vi "Particle Detection.vi"() -> ()   [LabVIEW 2014]
uses:
  <vilib>/userdefined/High Color/IMAQdx.ctl
  <vilib>/vision/driver/NI_Vision_Acquisition_Software.lvlib
  <vilib>/vision/NI_Vision_Development_Module.lvlib
panel:
  out "Before erosion":T1(plugin-control)
  out "Number of Particles after":i32
  out "After erosions":T1(plugin-control)
  in  "milliseconds to wait":u32
  out "Original":T1(plugin-control)
  in  "Number of Erosion":i32=2
  out "Number of Particles before":i32
  in  "stop":bool
  out "error out":errorcluster
  in  "error in (no error)":errorcluster
  in  "Image Name":string="webcam"
  in  "Session In":T2="cam0"
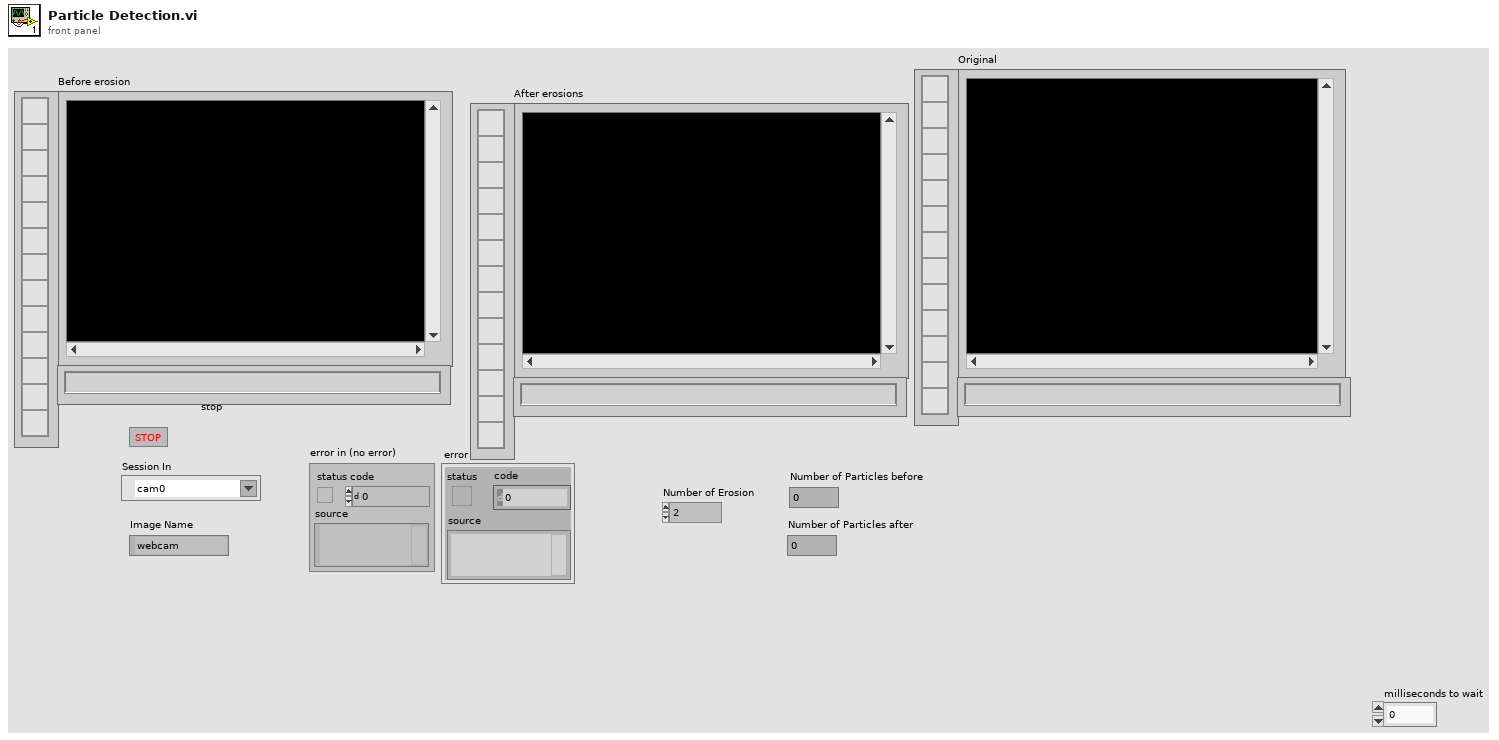
[diagram p1: front panel]
types:
  T1 = typedef "IMAQ Image.ctl" = refnum<image>
  T2 = typedef "IMAQdx.ctl" = refnum<k21>
  T3 = typedef "Image Type" = u32
  T4 = typedef "Particle Parameters" = i32
  T5 = cluster{"Numeric":dbl, "Numeric":dbl, "Numeric":dbl, "Numeric":dbl}
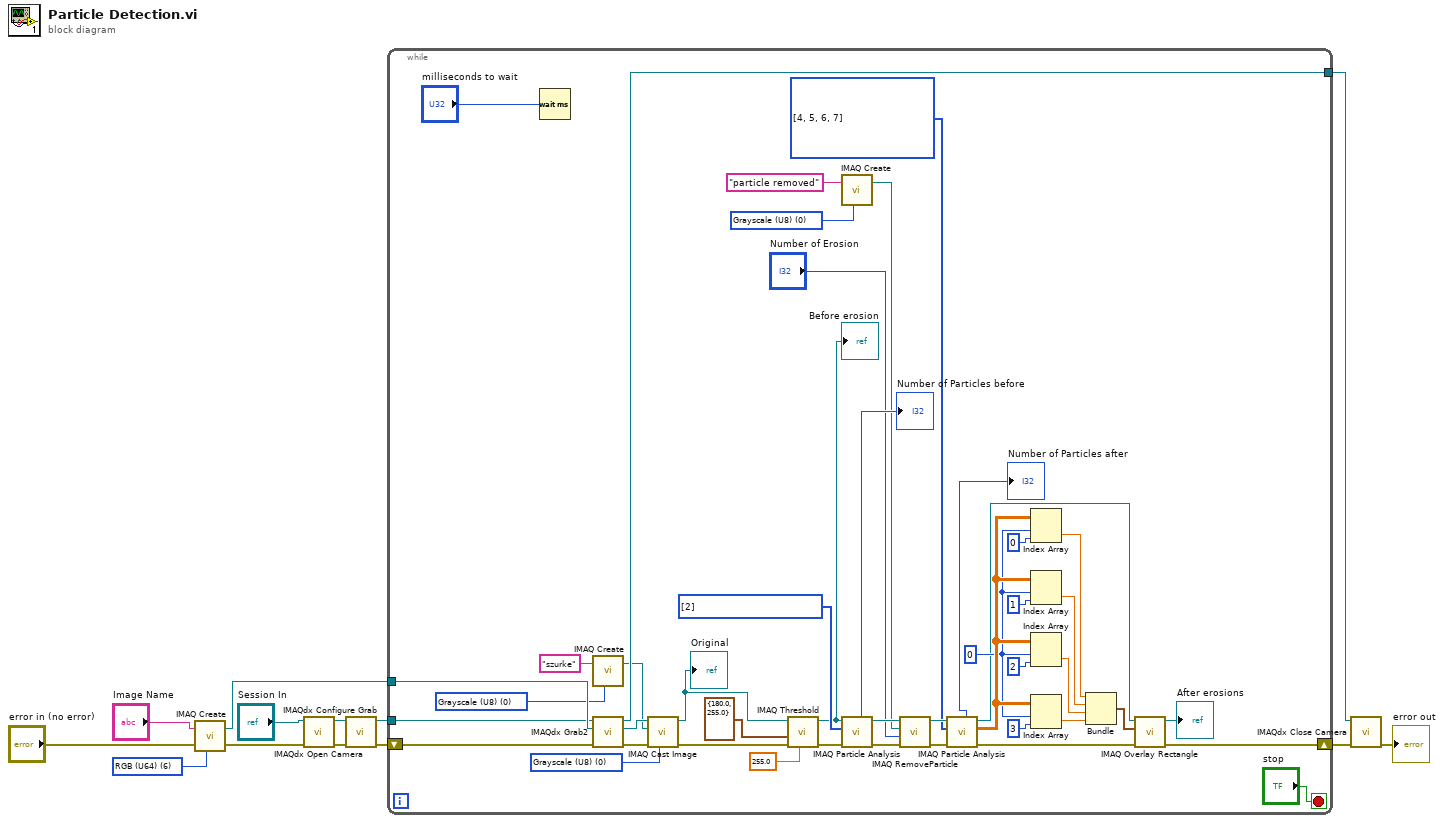
[diagram p0: block diagram]
diagram:
  w10 = T3 6 items=["Grayscale (U8)", "Grayscale (I16)", "Grayscale (SGL)", "Complex (CSG)", "RGB (U32)", "HSL (U32)", "RGB (U64)", "Grayscale (U16)"] ("Image Type")
  n1 = call "IMAQ Create"("Image Name"="Image Name", "Image Type"=w10, "error in (no error)"="error in (no error)") -> ("New Image"=w9:T1, "error out"=w7:errorcluster)  [unwired: 2 in]
  n2 = call <vilib>:"IMAQdx Open Camera.vi"("error in"=w7, "Session In"="Session In") -> ("error out"=w2:errorcluster, "Session Out"=w4:T2)  [unwired: 8 in]
  n3 = call <vilib>:"IMAQdx Configure Grab.vi"("error in"=w2, "Session In"=w4) -> ("error out"=w1:errorcluster, "Session Out"=w3:T2)  [unwired: 8 in]
  n4 = while {
    tunnel: w9 -> [w58]
    shift-right: [w15] -> w13
    shift-left: w1 -> [w55]
    tunnel: w3 -> [w56]
    tunnel: [w54] -> w11
    stop <- "stop" stop-if-true
    w27 = 0 ("index (row)")
    w29 = T4[] [4, 5, 6, 7] items=["Center of Mass X", "Center of Mass Y", "First Pixel X", "First Pixel Y", "Bounding Rect Left", "Bounding Rect Top", "Bounding Rect Right", "Bounding Rect Bottom", "Max Feret Diameter Start X", "Max Feret Diameter Start Y", "Max Feret Diameter End X", "Max Feret Diameter End Y", "Max Horiz. Segment Length Left", "Max Horiz. Segment Length Right", "Max Horiz. Segment Length Row", "-", "Bounding Rect Width", "Bounding Rect Height", "Bounding Rect Diagonal", "Perimeter", "Convex Hull Perimeter", "Holes' Perimeter", "Max Feret Diameter", "Equivalent Ellipse Major Axis", "Equivalent Ellipse Minor Axis", "Equivalent Ellipse Minor Axis (Feret)", "Equivalent Rect Long Side", "Equivalent Rect Short Side", "Equivalent Rect Diagonal", "Equivalent Rect Short Side (Feret)", "Average Horiz. Segment Length", "Average Vert. Segment Length", "Hydraulic Radius", "Waddel Disk Diameter", "-", "Area", "Holes' Area", "Particle & Holes' Area", "Convex Hull Area", "Image Area", "-", "Number of Holes", "Number of Horiz. Segments", "Number of Vert. Segments", "-", "Orientation", "Max Feret Diameter Orientation", "-", "% Area/Image Area", "% Area/(Particle & Holes' Area)", "Ratio of Equivalent Ellipse Axes", "Ratio of Equivalent Rect Sides", "-", "Elongation Factor", "Compactness Factor", "Heywood Circularity Factor", "Type Factor", "-", "Sum X", "Sum Y", "Sum XX", "Sum XY", "Sum YY", "Sum XXX", "Sum XXY", "Sum XYY", "Sum YYY", "-", "Moment of Inertia XX", "Moment of Inertia XY", "Moment of Inertia YY", "Moment of Inertia XXX", "Moment of Inertia XXY", "Moment of Inertia XYY", "Moment of Inertia YYY", "Norm. Moment of Inertia XX", "Norm. Moment of Inertia XY", "Norm. Moment of Inertia YY", "Norm. Moment of Inertia XXX", "Norm. Moment of Inertia XXY", "Norm. Moment of Inertia XYY", "Norm. Moment of Inertia YYY", "Hu Moment 1", "Hu Moment 2", "Hu Moment 3", "Hu Moment 4", "Hu Moment 5", "Hu Moment 6", "Hu Moment 7"] ("Pixel Measurements")
    w36 = T3 0 items=["Grayscale (U8)", "Grayscale (I16)", "Grayscale (SGL)", "Complex (CSG)", "RGB (U32)", "HSL (U32)", "RGB (U64)", "Grayscale (U16)"] ("Image Type")
    w37 = T3 0 items=["Grayscale (U8)", "Grayscale (I16)", "Grayscale (SGL)", "Complex (CSG)", "RGB (U32)", "HSL (U32)", "RGB (U64)", "Grayscale (U16)"] ("Image Type")
    w48 = T4[] [2] items=["Center of Mass X", "Center of Mass Y", "First Pixel X", "First Pixel Y", "Bounding Rect Left", "Bounding Rect Top", "Bounding Rect Right", "Bounding Rect Bottom", "Max Feret Diameter Start X", "Max Feret Diameter Start Y", "Max Feret Diameter End X", "Max Feret Diameter End Y", "Max Horiz. Segment Length Left", "Max Horiz. Segment Length Right", "Max Horiz. Segment Length Row", "-", "Bounding Rect Width", "Bounding Rect Height", "Bounding Rect Diagonal", "Perimeter", "Convex Hull Perimeter", "Holes' Perimeter", "Max Feret Diameter", "Equivalent Ellipse Major Axis", "Equivalent Ellipse Minor Axis", "Equivalent Ellipse Minor Axis (Feret)", "Equivalent Rect Long Side", "Equivalent Rect Short Side", "Equivalent Rect Diagonal", "Equivalent Rect Short Side (Feret)", "Average Horiz. Segment Length", "Average Vert. Segment Length", "Hydraulic Radius", "Waddel Disk Diameter", "-", "Area", "Holes' Area", "Particle & Holes' Area", "Convex Hull Area", "Image Area", "-", "Number of Holes", "Number of Horiz. Segments", "Number of Vert. Segments", "-", "Orientation", "Max Feret Diameter Orientation", "-", "% Area/Image Area", "% Area/(Particle & Holes' Area)", "Ratio of Equivalent Ellipse Axes", "Ratio of Equivalent Rect Sides", "-", "Elongation Factor", "Compactness Factor", "Heywood Circularity Factor", "Type Factor", "-", "Sum X", "Sum Y", "Sum XX", "Sum XY", "Sum YY", "Sum XXX", "Sum XXY", "Sum XYY", "Sum YYY", "-", "Moment of Inertia XX", "Moment of Inertia XY", "Moment of Inertia YY", "Moment of Inertia XXX", "Moment of Inertia XXY", "Moment of Inertia XYY", "Moment of Inertia YYY", "Norm. Moment of Inertia XX", "Norm. Moment of Inertia XY", "Norm. Moment of Inertia YY", "Norm. Moment of Inertia XXX", "Norm. Moment of Inertia XXY", "Norm. Moment of Inertia XYY", "Norm. Moment of Inertia YYY", "Hu Moment 1", "Hu Moment 2", "Hu Moment 3", "Hu Moment 4", "Hu Moment 5", "Hu Moment 6", "Hu Moment 7"] ("Pixel Measurements")
    w52 = T3 0 items=["Grayscale (U8)", "Grayscale (I16)", "Grayscale (SGL)", "Complex (CSG)", "RGB (U32)", "HSL (U32)", "RGB (U64)", "Grayscale (U16)"] ("Image Type")
    n5 = Wait (ms)(milliseconds to wait="milliseconds to wait") -> ()  [unwired: 1 out]
    n6 = call "IMAQ Create"("Image Name"="szurke", "Image Type"=w37) -> ("New Image"=w38:T1)  [unwired: 3 in, 1 out]
    n7 = call <vilib>:"IMAQdx Grab2.vi"("error in"=w55, "Image In"=w58, "Session In"=w56) -> ("error out"=w53:errorcluster, "Image Out"=w39:T1, "Session Out"=w54:T2)  [unwired: 5 in, 1 out]
    n8 = call "IMAQ Cast Image"("Image Type"=w52, "error in (no error)"=w53, "Image Dst"=w38, "Image Src"=w39) -> ("error out"=w49:errorcluster, "Image Dst Out"=w34:T1)  [unwired: 6 in]
    "Original" <- w34
    n9 = call "IMAQ Threshold"("Replace Value"=sgl 255.0, "error in (no error)"=w49, "Range"=cluster{"Lower value":sgl, "Upper value":sgl} {"Lower value"=180.0, "Upper value"=255.0}, "Image Src"=w34) -> ("error out"=w46:errorcluster, "Image Dst Out"=w30:T1)  [unwired: 6 in]
    "Before erosion" <- w30
    n10 = call "IMAQ Create"("Image Name"="particle removed", "Image Type"=w36) -> ("New Image"=w42:T1)  [unwired: 3 in, 1 out]
    n11 = call "IMAQ Particle Analysis"("error in (no error)"=w46, "Pixel Measurements"=w48, "Image"=w30) -> ("error out"=w43:errorcluster, "Image Out (duplicate)"=w45:T1, "Number of Particles"=→"Number of Particles before":i32)  [unwired: 3 in, 3 out]
    n12 = call "IMAQ RemoveParticle"("error in (no error)"=w43, "Number of Erosion"="Number of Erosion", "Image Dst"=w42, "Image Src"=w45) -> ("error out"=w32:errorcluster, "Image Dst Out"=w31:T1)  [unwired: 6 in]
    n13 = call "IMAQ Particle Analysis"("error in (no error)"=w32, "Pixel Measurements"=w29, "Image"=w31) -> ("error out"=w14:errorcluster, "Particle Measurements (Pixels)"=w28:dbl[][], "Image Out (duplicate)"=w16:T1, "Number of Particles"=→"Number of Particles after":i32)  [unwired: 3 in, 2 out]
    n14 = Index Array(array=w28, index (row)=w27, index (col)=0 ("disabled index (col)")) -> (element=w22:dbl)
    n15 = Index Array(array=w28, index (row)=w27, index (col)=1 ("disabled index (col)")) -> (element=w21:dbl)
    n16 = Index Array(array=w28, index (row)=w27, index (col)=2 ("disabled index (col)")) -> (element=w20:dbl)
    n17 = Index Array(array=w28, index (row)=w27, index (col)=3 ("disabled index (col)")) -> (element=w19:dbl)
    n18 = Bundle("Numeric"=w22, "Numeric"=w21, "Numeric"=w20, "Numeric"=w19) -> (w18:T5)  [unwired: 1 in]
    n19 = call "IMAQ Overlay Rectangle"("error in (no error)"=w14, "Rectangle"=w18, "Image"=w16) -> ("error out"=w15:errorcluster, "Image Out"=→"After erosions":T1)  [unwired: 7 in]
  }
  n20 = call <vilib>:"IMAQdx Close Camera.vi"("error in"=w13, "Session In"=w11) -> ("error out"=→"error out":errorcluster)  [unwired: 9 in]
